vi "UpdatePrice.vi"(8 "error in (no error)":errorcluster, 10 "Time Stamp":timestamp, 11 "USD":dbl) -> (0 "error out":errorcluster)   [LabVIEW 2017, in "UI.lvlib"]
doc: "Write data to main coms q for module (generic)"
uses:
  ctl/MainData.ctl
  ctl/MainStates.ctl
  ctl/Price.ctl
  UI.lvlib
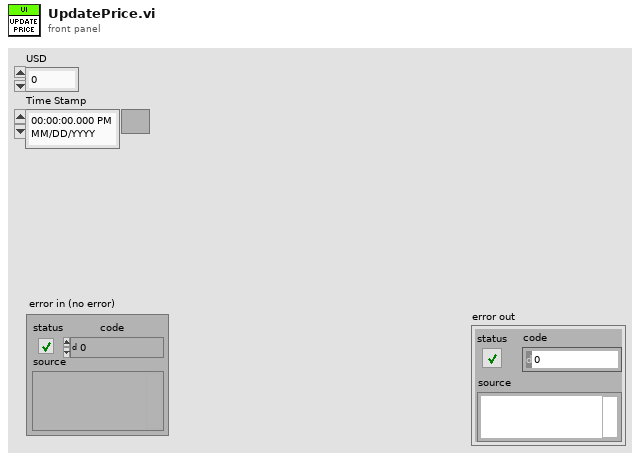
[diagram p1: front panel]
types:
  T1 = typedef "UI.lvlib/MainStates.ctl" = enum16{"Timeout", "Error", "Exit", "Init", "UpdatePrice", "CloseAll"}
  T2 = typedef "UI.lvlib/Price.ctl" = cluster{"USD":dbl, "Time Stamp":timestamp}
  T3 = typedef "UI.lvlib/MainData.ctl" = cluster{"State":T1, "Variant":variant}
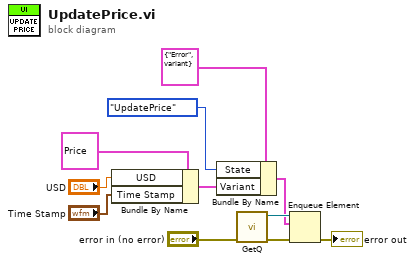
[diagram p0: block diagram]
diagram:
  n1 = Bundle By Name(cluster=T2 {"USD"=0.0, "Time Stamp"=timestamp(0 s since 1904-01-01)} ("Price"), "USD"="USD", "Time Stamp"="Time Stamp") -> (w4:T2)
  n2 = Bundle By Name(cluster=T3 {"State"=enum."Error", "Variant"=variant} ("Data"), "State"=MainStates."UpdatePrice", "Variant"=w4) -> (w7:T3)
  n3 = call "GetQ.vi"("error in (no error)"="error in (no error)") -> ("error out"=w10:errorcluster, "Q out"=w11:refnum<queue>)  [unwired: 9 in]
  n4 = Enqueue Element(queue=w11, element=w7, error in (no error)=w10) -> (error out=→"error out":errorcluster)  [unwired: 1 in, 2 out]
